vi "ExposeOnGetValue.vi"(8 "Requires Response":bool, 9 "Message":T2 {"Message Type" items=["Error"=1, "Warning"=2, "Create"=4, "Destroy"=8, "Invoke"=16, "Get"=32, "Set"=64, "Response"=128]}, 10 "HandlerID":string, 11 "Expose Info":T1) -> (3 "Response":variant)   [LabVIEW 2017]
uses:
  ExposeMessage.ctl
  Events/ExposeMessageType.ctl
  Mapper/ExposeObjectMapNamepathData.ctl
  Mapper/ExposeMapperDataTypeEnum.ctl
  Mapper/ExposeObjectMapContainerTypeEnum.ctl
  ExposeInfo.ctl
  C:/Code/CMCryoSysCode/Expose/COM/CSCom/CSCom/bin/Release/CSCom.dll
  COM/CSCom/CSCom/bin/Release/CSCom.dll
  ExposeDataType.ctl
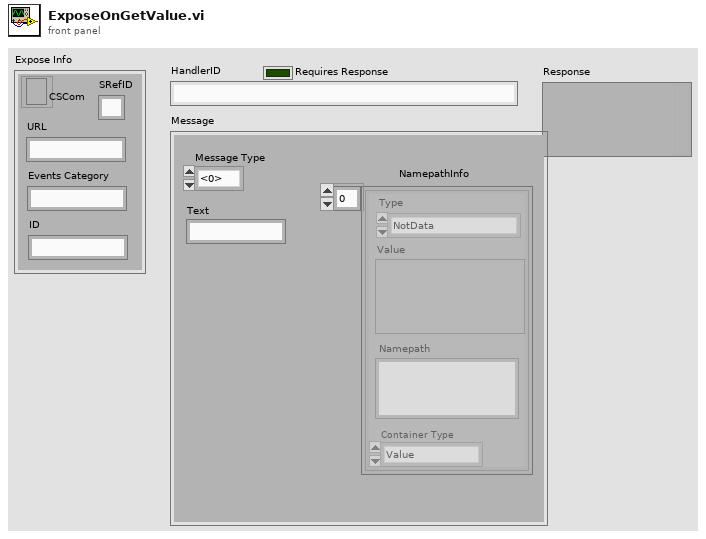
[diagram p1: front panel]
types:
  T1 = typedef "ExposeInfo.ctl" = cluster{"CSCom":refnum<k24>, "URL":string, "Events Category":string, "ID":string, "SRefID":string}
  T2 = typedef "ExposeMessage.ctl" = cluster{"Message Type":T3, "Text":string, "NamepathInfo":T4[]}
  T3 = typedef "ExposeMessageType.ctl" = i32
  T4 = typedef "ExposeObjectMapNamepathData.ctl" = cluster{"Type":T5, "Value":variant, "Namepath":string, "Container Type":T6}
  T5 = typedef "ExposeMapperDataTypeEnum.ctl" = enum16{"NotData", "int8", "byte", "int16", "uint16", "int32", "uint32", "int64", "uint64", "Single", "Double", "String", "Boolean", "Container"}
  T6 = typedef "ExposeObjectMapContainerTypeEnum.ctl" = enum16{"Value", "Array", "Waveform", "NetContainer"}
  T7 = typedef "ExposeDataType.ctl" = cluster{"Values":variant, "ParameterBindingInfo":variant}
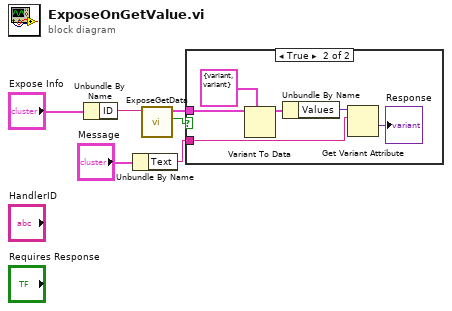
[diagram p0: block diagram]
diagram:
  n1 = Unbundle By Name("Expose Info") -> ("ID"=w4:string)
  n2 = Unbundle By Name("Message") -> ("Text"=w1:string)
  n3 = call "ExposeGetData.vi"("ExposeID"=w4) -> ("isnew?"=w3:bool, "ExposeDataType"=w2:T7)  [unwired: 9 in]
  n4 = case shown="True" w3 {
    tunnel: w2 -> [_ w11]
    tunnel: w1 -> [_ w8]
    frame False {
    }
    frame True {
      n5 = Variant To Data(type=T7 {"Values"=variant, "ParameterBindingInfo"=variant} ("ExposeDataType"), Variant=w11) -> (data=w10:T7)  [unwired: 1 in, 1 out]
      n6 = Unbundle By Name(w10) -> ("Values"=w9:variant)
      n7 = Get Variant Attribute(Variant=w9, name=w8) -> (value=→"Response":variant)  [unwired: 2 in, 3 out]
    }
  }
